vi "Send Communiation to Target.vi"(8 "error in":errorcluster, 9 "Data":string, 10 "Name":string="SendToCRIO", 11 "Program Data":T1={"Measurements"={"Channel 0"="Channel 0", "RMS 0"="RMS:", "Vp-p 0"="Vp-p:", "Freq 0"="Freq:", "Channel 1"="Channel 1", "RMS 1"="RMS:", "Vp-p 1"="Vp-p:", "Freq 1"="Freq:", "Cursors"="Channel 0", "C1"="Channel 0", "C2"="Channel 0", "dT"="Channel 0"}, "C1"={"Name"="", "X"=0.0, "Y"=0.0}, "C2"={"Name"="", "X"=0.0, "Y"=0.0}, "Com"={"Connection Info"={"connection ID"=refnum, "meta data"=[]}, "Connected?"=FALSE, "IP"=""}, "Continuous?"=FALSE, "Scope Data"={"AI0"=[], "AI1"=[]}, "Wave Parameters"={"Frequency (Hz)"=5.0, "Phase offset (deg)"=0.0, "Vpeak (V)"=5.0, "Offset (V)"=0.0, "Waveform"=enum."Sine", "Channel"=enum."CH0"}, "Acquire?"=FALSE, "Measure Ref"=refnum, "CH0"={"Channel"=enum."AI 0", "Enable"=FALSE, "Volts/Div"=0, "Vertical Position (Div)"=0.0}, "CH1"={"Channel"=enum."AI 0", "Enable"=FALSE, "Volts/Div"=0, "Vertical Position (Div)"=0.0}, "CH0 Params"={"V/Div"=0.0, "Units"=""}, "CH1 Params"={"V/Div"=0.0, "Units"=""}, "Time"={"Time/Div"=0.0}, "dT"=0.0, "FGen"={"Offset (V)"=0.0, "Enable Sweep"=FALSE, "Start Frequency (Hz)"=0.0, "Stop Frequency (Hz)"=0.0, "Step (Hz)"=0.0, "Step Interval (ms)"=0.0, "Current Freq (Hz)"=0.0, "Run"=FALSE}} {"Time"."Time/Div" min=0.0 max=16.0 step=1.0 scale=0.0..12.0; "CH1"."Vertical Position (Div)" min=-5.0 max=5.0 step=0.1 scale=-5.0..5.0; "CH1"."Volts/Div" min=0 max=8 step=1 scale=0.0..8.0; "CH0"."Vertical Position (Div)" min=-5.0 max=5.0 step=0.1 scale=-5.0..5.0; "CH0"."Volts/Div" min=0 max=8 step=1 scale=0.0..8.0; "Wave Parameters"."Phase offset (deg)" format="%#_6p"; "Wave Parameters"."Frequency (Hz)" format="%#_6p"}) -> (0 "error out":errorcluster, 3 "Program Data Out":T1={"Measurements"={"Channel 0"="Channel 0", "RMS 0"="RMS:", "Vp-p 0"="Vp-p:", "Freq 0"="Freq:", "Channel 1"="Channel 1", "RMS 1"="RMS:", "Vp-p 1"="Vp-p:", "Freq 1"="Freq:", "Cursors"="Channel 0", "C1"="Channel 0", "C2"="Channel 0", "dT"="Channel 0"}, "C1"={"Name"="", "X"=0.0, "Y"=0.0}, "C2"={"Name"="", "X"=0.0, "Y"=0.0}, "Com"={"Connection Info"={"connection ID"=refnum, "meta data"=[]}, "Connected?"=FALSE, "IP"=""}, "Continuous?"=FALSE, "Scope Data"={"AI0"=[], "AI1"=[]}, "Wave Parameters"={"Frequency (Hz)"=5.0, "Phase offset (deg)"=0.0, "Vpeak (V)"=5.0, "Offset (V)"=0.0, "Waveform"=enum."Sine", "Channel"=enum."CH0"}, "Acquire?"=FALSE, "Measure Ref"=refnum, "CH0"={"Channel"=enum."AI 0", "Enable"=FALSE, "Volts/Div"=0, "Vertical Position (Div)"=0.0}, "CH1"={"Channel"=enum."AI 0", "Enable"=FALSE, "Volts/Div"=0, "Vertical Position (Div)"=0.0}, "CH0 Params"={"V/Div"=0.0, "Units"=""}, "CH1 Params"={"V/Div"=0.0, "Units"=""}, "Time"={"Time/Div"=0.0}, "dT"=0.0, "FGen"={"Offset (V)"=0.0, "Enable Sweep"=FALSE, "Start Frequency (Hz)"=0.0, "Stop Frequency (Hz)"=0.0, "Step (Hz)"=0.0, "Step Interval (ms)"=0.0, "Current Freq (Hz)"=0.0, "Run"=FALSE}} {"Time"."Time/Div" min=0.0 max=16.0 step=1.0 scale=0.0..12.0; "CH1"."Vertical Position (Div)" min=-5.0 max=5.0 step=0.1 scale=-5.0..5.0; "CH1"."Volts/Div" min=0 max=8 step=1 scale=0.0..8.0; "CH0"."Vertical Position (Div)" min=-5.0 max=5.0 step=0.1 scale=-5.0..5.0; "CH0"."Volts/Div" min=0 max=8 step=1 scale=0.0..8.0; "Wave Parameters"."Phase offset (deg)" format="%#_6p"; "Wave Parameters"."Frequency (Hz)" format="%#_6p"})   [LabVIEW 2021]
uses:
  Controls/Program Data.ctl
  Controls/Measurements.ctl
  Controls/Channel Measurement String Control.ctl
  Controls/Cursor Info.ctl
  Controls/Communication Cluster.ctl
  <vilib>/NI/STM/TCP/TCP Connection Info.ctl
  <vilib>/NI/STM/SubVIs/MetaDataElement.ctl
  Scope Data.ctl
  Program Files (x86)/National Instruments/LabVIEW 2021/ProjectTemplates/Source/myRIO/Oscilloscope/myRIO v1.1/Real-Time/Controls/Wave Parameters.ctl
  Program Files (x86)/National Instruments/LabVIEW 2021/ProjectTemplates/Source/myRIO/Oscilloscope/myRIO v1.1/Real-Time/Controls/Waveform Enum.ctl
  Program Files (x86)/National Instruments/LabVIEW 2021/ProjectTemplates/Source/myRIO/Oscilloscope/myRIO v1.1/Real-Time/Controls/Channel Selector.ctl
  Controls/Channel Settings.ctl
  Controls/Analog Input Selector.ctl
  Controls/Knob.ctl
  Controls/Vertical Position.ctl
  Controls/Channel Parameters.ctl
  Controls/Time Selector.ctl
  Controls/Time Knob.ctl
  Controls/FGen Desktop Configuration.ctl
  <vilib>/NI/STM/TCP/Write Message (TCP).vi
  <vilib>/NI/STM/NI STM.lvlib
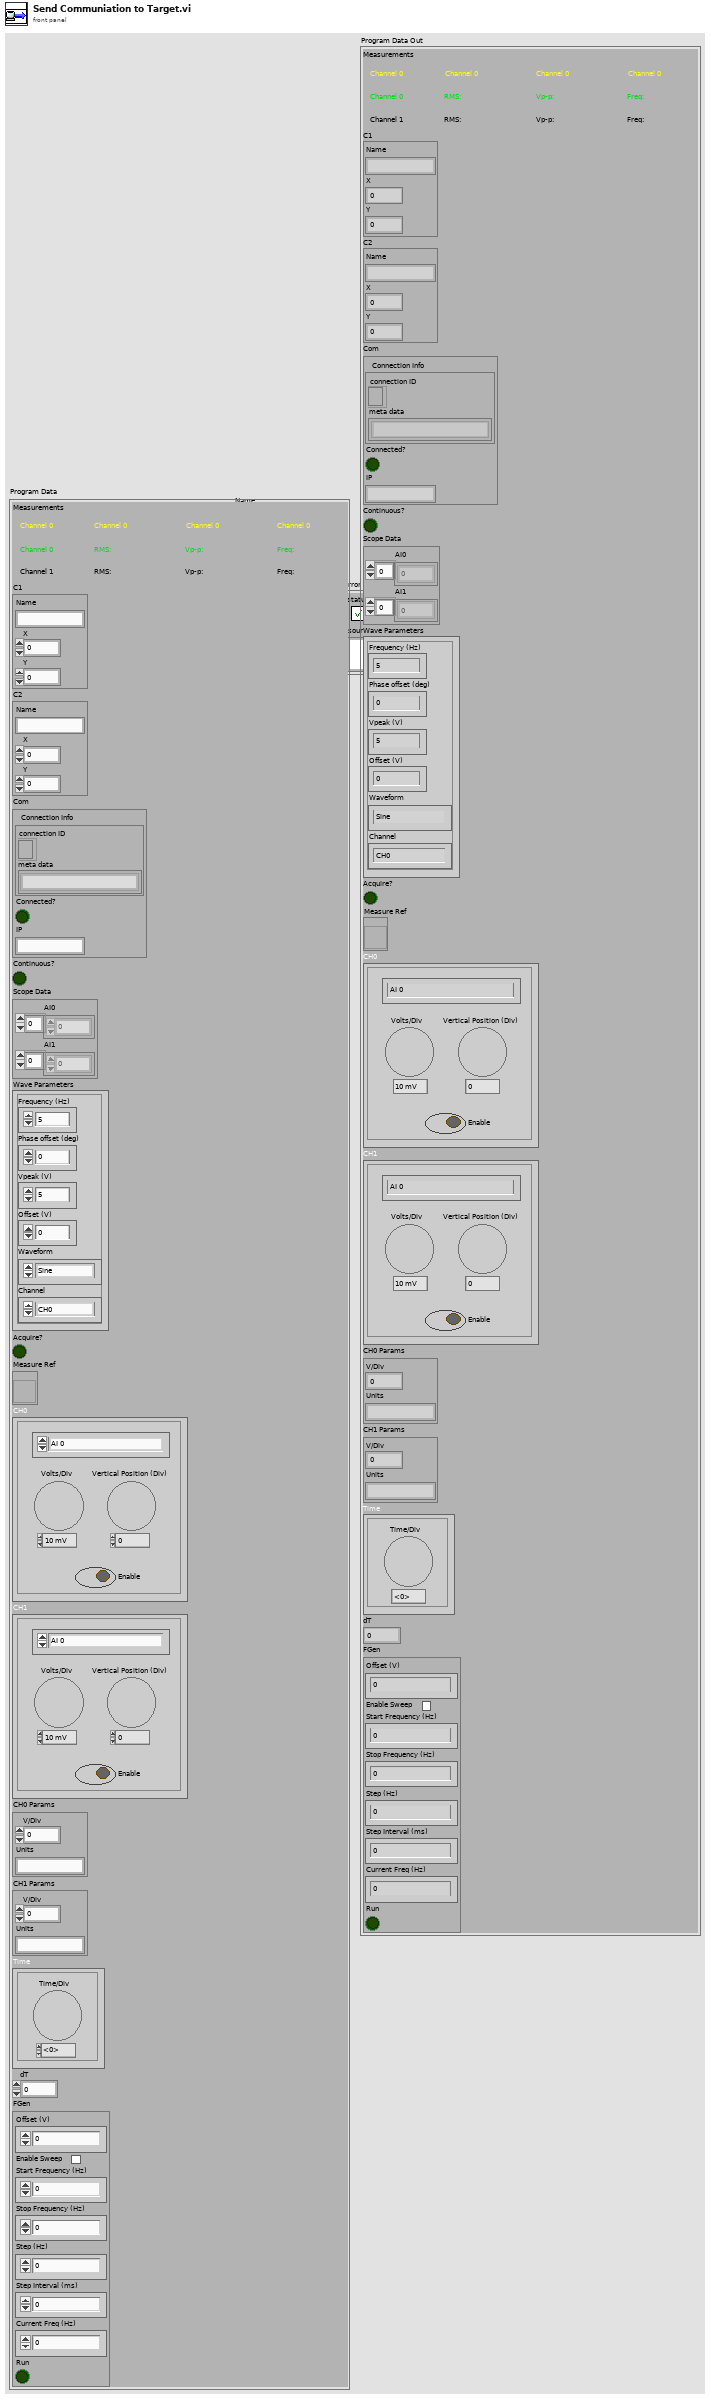
[diagram p1: front panel]
types:
  T1 = typedef "Program Data.ctl" = cluster{"Measurements":T2, "C1":T4, "C2":T4, "Com":T5, "Continuous?":bool, "Scope Data":T8, "Wave Parameters":T9, "Acquire?":bool, "Measure Ref":refnum<vi>, "CH0":T12, "CH1":T12, "CH0 Params":T16, "CH1 Params":T16, "Time":T17, "dT":dbl, "FGen":T19}
  T2 = typedef "Measurements.ctl" = cluster{"Channel 0":T3, "RMS 0":T3, "Vp-p 0":T3, "Freq 0":T3, "Channel 1":T3, "RMS 1":T3, "Vp-p 1":T3, "Freq 1":T3, "Cursors":T3, "C1":T3, "C2":T3, "dT":T3}
  T3 = typedef "Channel Measurement String Control.ctl" = string
  T4 = typedef "Cursor Info.ctl" = cluster{"Name":string, "X":dbl, "Y":dbl}
  T5 = typedef "Communication Cluster.ctl" = cluster{"Connection Info":T6, "Connected?":bool, "IP":string}
  T6 = typedef "NI STM.lvlib/TCP Connection Info.ctl" = cluster{"connection ID":refnum<k5>, "meta data":T7[]}
  T7 = typedef "NI STM.lvlib/MetaDataElement.ctl" = string
  T8 = typedef "Scope Data.ctl" = cluster{"AI0":dbl[], "AI1":dbl[]}
  T9 = typedef "Wave Parameters.ctl" = cluster{"Frequency (Hz)":dbl, "Phase offset (deg)":dbl, "Vpeak (V)":dbl, "Offset (V)":dbl, "Waveform":T10, "Channel":T11}
  T10 = typedef "Waveform Enum.ctl" = enum16{"Sine", "Square"}
  T11 = typedef "Channel Selector.ctl" = enum16{"CH0", "CH1"}
  T12 = typedef "Channel Settings.ctl" = cluster{"Channel":T13, "Enable":bool, "Volts/Div":T14, "Vertical Position (Div)":T15}
  T13 = typedef "Analog Input Selector.ctl" = enum16{"AI 0", "AI 1"}
  T14 = typedef "Knob.ctl" = i32
  T15 = typedef "Vertical Position.ctl" = dbl
  T16 = typedef "Channel Parameters.ctl" = cluster{"V/Div":dbl, "Units":string}
  T17 = typedef "Time Selector.ctl" = cluster{"Time/Div":T18}
  T18 = typedef "Time Knob.ctl" = dbl
  T19 = typedef "FGen Desktop Configuration.ctl" = cluster{"Offset (V)":dbl, "Enable Sweep":bool, "Start Frequency (Hz)":dbl, "Stop Frequency (Hz)":dbl, "Step (Hz)":dbl, "Step Interval (ms)":dbl, "Current Freq (Hz)":dbl, "Run":bool}
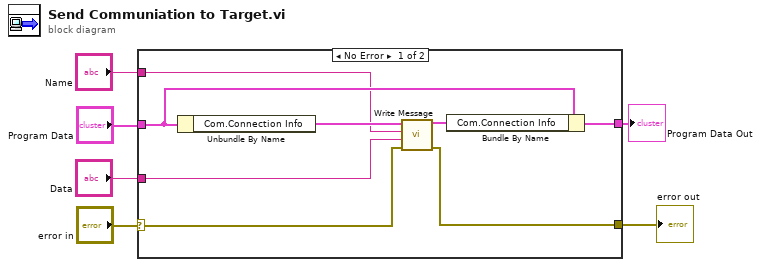
[diagram p0: block diagram]
diagram:
  n1 = case shown="No Error" "error in" {
    selector: "error in" -> [w8 w15]
    tunnel: "Program Data" -> [w13 w16]
    tunnel: [w11 w15] -> w3
    tunnel: [w10 w16] -> w1
    tunnel: "Name" -> [w9 _]
    tunnel: "Data" -> [w7 _]
    frame No Error {
      n2 = Unbundle By Name(w13) -> ("Com.Connection Info"=w14:T6)
      n3 = call-poly <vilib>:"Write Message.vi"("error in"=w8, "data"=w7, "name"=w9, "connection info in"=w14) -> ("error out"=w11:errorcluster, "connection info out"=w12:T6)  [unwired: 1 in, 5 out]
      n4 = Bundle By Name(cluster=w13, "Com.Connection Info"=w12) -> (w10:T1)
    }
    frame Error {
    }
  }
  "error out" <- w3
  "Program Data Out" <- w1
